vi "Delete Profile.vi"(8 "error in (no error)":errorcluster, 11 "SSID":string) -> (0 "error out":errorcluster, 3 "Feedback":string)   [LabVIEW 2017]
doc: "Removes a WLAN profile from one or multiple interfaces."
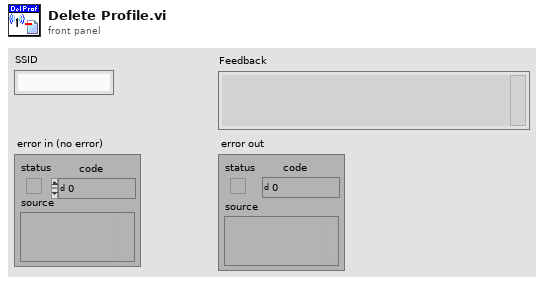
[diagram p1: front panel]
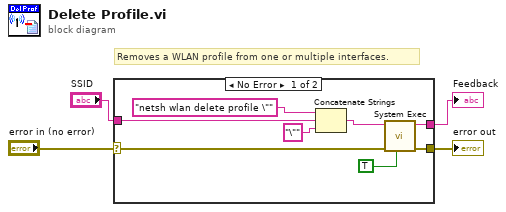
[diagram p0: block diagram]
diagram:
  # "Removes a WLAN profile from one or multiple interfaces."
  n1 = case shown="No Error" "error in (no error)" {
    selector: "error in (no error)" -> [w12 w13]
    tunnel: [w11 w13] -> w3
    tunnel: "SSID" -> [w9 _]
    tunnel: [w5 _] -> w1
    frame No Error {
      n2 = Concatenate Strings("netsh wlan delete profile \"" ("string"), w9, "\"" ("string")) -> (w6:string)
      n3 = call <vilib>:"System Exec.vi"("run minimized? (F)"=TRUE, "error in (no error)"=w12, "command line"=w6) -> ("error out"=w11:errorcluster, "standard output"=w5:string)  [unwired: 5 in, 2 out]
    }
    frame Error {
    }
  }
  "error out" <- w3
  "Feedback" <- w1
